vi "neuron.vi"(8 "opinons":dbl[](array[numeric]), 11 "inputs":dbl[][](array[numeric])) -> (2 "output":dbl[](array[numeric]))   [LabVIEW 2014]
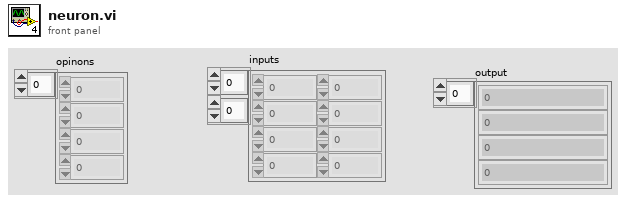
[diagram p1: front panel]
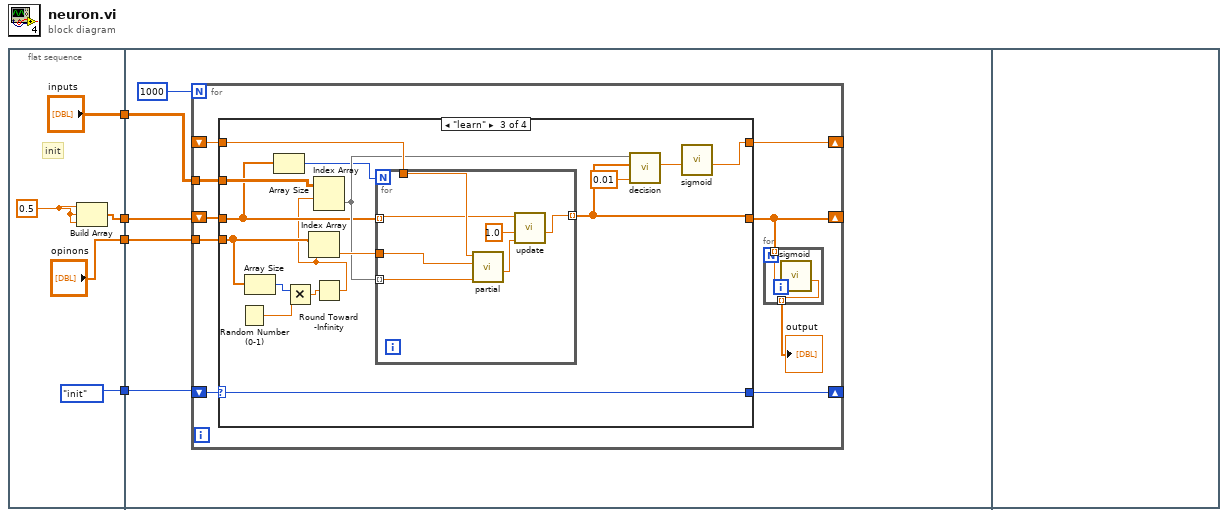
[diagram p0: block diagram]
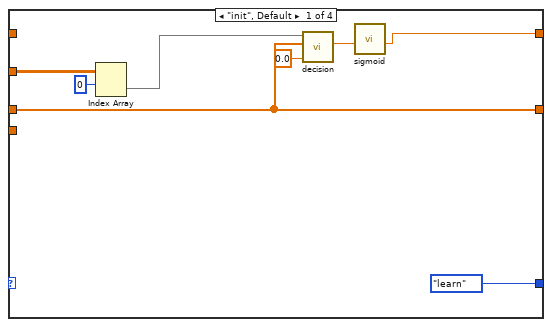
[diagram p2: hidden frame]
diagram:
  n1 = flat-sequence {
    tunnel: [enum16{"init", "idle", "learn", "estimate"}."init"] -> w4
    tunnel: [w8] -> w3
    tunnel: ["inputs"] -> w2
    tunnel: ["opinons"] -> w1
    tunnel: w4 -> [w14]
    tunnel: w3 -> [w11]
    tunnel: w2 -> [w10]
    tunnel: w1 -> [w12]
    frame #0 {
      w5 = 0.5 ("element")
      # "init"
      n2 = Build Array(w5, w5, w5) -> (w8:dbl[])
    }
    frame #1 {
      n3 = for {
        N: 1000 -> [_]
        shift-right: [w23] -> _
        shift-left: _ -> [w22]
        shift-right: [w21] -> _
        shift-left: w14 -> [w20]
        tunnel: w12 -> [w19]
        shift-right: [w15] -> _
        shift-left: w11 -> [w18]
        tunnel: w10 -> [w17]
        n4 = case shown="\"learn\"" w20 {
          selector: w20 -> [_ w34 w52 w60]
          tunnel: [w32 w35 w41 w62] -> w23
          tunnel: w22 -> [_ w35 w51 w62]
          tunnel: [enum16{"init", "idle", "learn", "estimate"}."learn" w34 w52 w60] -> w21
          tunnel: w18 -> [w28 w36 w39 w61]
          tunnel: w17 -> [w29 _ w47 _]
          tunnel: w19 -> [_ _ w48 _]
          tunnel: [w28 w36 w42 w61] -> w15
          frame "init", Default {
            n5 = Index Array(array=w29, index (row)=0) -> (element=w26:dbl[])  [unwired: 1 in]
            n6 = call "decision.vi"("offset"=0.0, "weights"=w28, "inputs"=w26) -> ("decision"=w33:dbl)  [unwired: 8 in]
            n7 = call "sigmoid.vi"("t"=w33) -> ("S(t)"=w32:dbl)  [unwired: 10 in]
          }
          frame "idle" {
          }
          frame "learn" {
            n8 = Random Number (0-1)() -> (number: 0 to 1=w49:dbl)
            n9 = Array Size(array=w48) -> (size(s)=w50:i32)
            n10 = Array Size(array=w39) -> (size(s)=w40:i32)
            n11 = Multiply(x=w50, y=w49) -> (x*y=w38:dbl)
            n12 = Round Toward -Infinity(1:w38) -> (0:w37:dbl)
            n13 = Index Array(array=w48, index=w37) -> (element=w46:dbl)
            n14 = Index Array(array=w47, index (row)=w37) -> (element=w43:dbl[])  [unwired: 1 in]
            n15 = for {
              N: w40 -> [_]
              tunnel: w51 -> [w57]
              tunnel: w39 -> [w56] mode=indexing
              tunnel: [w55] -> w42 mode=indexing
              tunnel: w43 -> [w54] mode=indexing
              tunnel: w46 -> [w53]
              n16 = call "partial.vi"("input"=w54, "opinon"=w53, "sigmoid g(~)"=w57) -> ("deltaX"=w58:dbl)  [unwired: 8 in]
              n17 = call "update.vi"("deltaX"=w58, "Alpha"=1.0, "X"=w56) -> ("X'"=w55:dbl)  [unwired: 8 in]
            }
            n18 = call "decision.vi"("offset"=0.01, "weights"=w42, "inputs"=w43) -> ("decision"=w45:dbl)  [unwired: 8 in]
            n19 = call "sigmoid.vi"("t"=w45) -> ("S(t)"=w41:dbl)  [unwired: 10 in]
          }
          frame "estimate" {
          }
        }
        n20 = for {
          tunnel: [w25] -> w16 mode=indexing
          tunnel: w15 -> [w24] mode=indexing
          n21 = call "sigmoid.vi"("t"=w24) -> ("S(t)"=w25:dbl)  [unwired: 10 in]
        }
        "output" <- w16
      }
    }
    frame #2 {
    }
  }
